vi "Engine In - Diesel - Sensors.vi"(0 "dt [sec]":sgl, 1 "ADCombo.Voltage [V]":sgl[](array[numeric]), 2 "ADCombo.Resistance [Ohm]":sgl[](array[numeric])) -> (8 "TDKBattV":sgl format="%0.2f", 9 "MAT [C]":sgl format="%0.2f", 10 "12VPulsBattV":sgl format="%0.2f", 11 "Oil Temp [C]":sgl, 12 "5VPulsBattV":sgl format="%0.2f", 13 "IAT [C]":sgl format="%0.2f", 14 "RailP [bar]":sgl format="%0.2f", 15 "ECT [C]":sgl format="%0.2f", 16 "Barometric Air Pressure [kPa]":sgl, 18 "Turbo Outlet Air Pressure [kPa]":sgl, 20 "MAP [kPa]":sgl format="%0.2f", 21 "Exhaust Manifold Pressure [kPa]":sgl, 22 "EGR DiffP [kPa]":sgl, 23 "Oil Pressure [kPa]":sgl, 24 "MAF [kg/hr]":sgl format="%0.2f", 25 "EGR Valve Position [%]":sgl, 26 "Pedal [%]":sgl format="%0.2f")   [LabVIEW 2015, in "ECS-RT.lvlib"]
uses:
  ECS-RT.lvlib
  <vilib>/ptbypt/NI_PtbyPt.lvlib
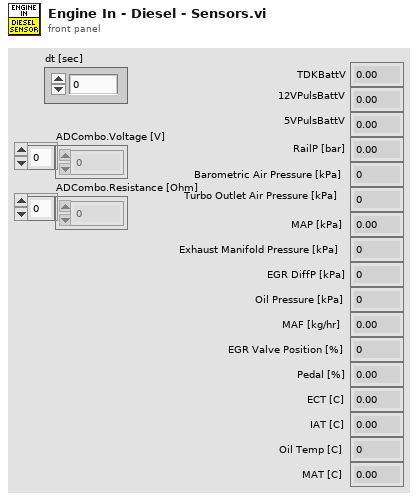
[diagram p1: front panel]
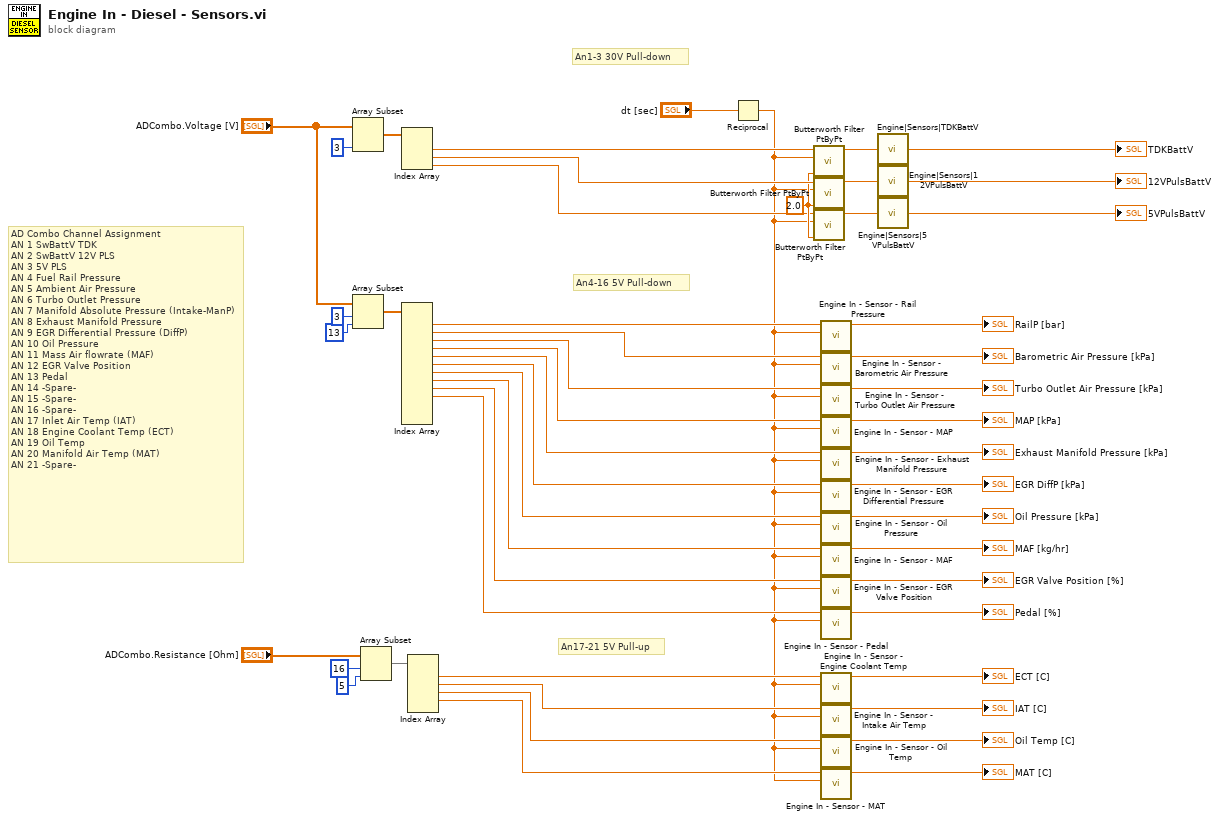
[diagram p0: block diagram]
diagram:
  w40 = 2.0 ("low cutoff freq: fl")
  # "An1-3 30V Pull-down"
  # "An17-21 5V Pull-up"
  # "An4-16 5V Pull-down"
  # "AD Combo Channel Assignment\nAN\t1\tSwBattV TDK\nAN\t2\tSwBattV 12V PLS\nAN\t3\t5V PLS\nAN\t4\tFuel Rail Pressure\nAN\t5\tAmbient Air Pressure\nAN\t6\tTurbo Outlet Pressure\nAN\t7\tManifold Absolute Pressure (Intake-ManP)\nAN\t8\tExhaust Manifold Pressure\nAN\t9\tEGR Differential Pressure (DiffP)\nAN\t10\tOil Pressure\nAN\t11\tMass Air flowrate (MAF)\nAN\t12\tEGR Valve Position\nAN\t13\tPedal\nAN\t14\t-Spare-\nAN\t15\t-Spare-\nAN\t16\t-Spare-\nAN\t17\tInlet Air Temp (IAT)\nAN\t18\tEngine Coolant Temp (ECT)\nAN\t19\tOil Temp\nAN\t20\tManifold Air Temp (MAT)\nAN\t21\t-Spare-"
  n1 = Array Subset(array="ADCombo.Voltage [V]", length=3) -> (w36:sgl[])  [unwired: 1 in]
  n2 = Array Subset(array="ADCombo.Voltage [V]", index=3, length=13) -> (w35:sgl[])
  n3 = Array Subset(array="ADCombo.Resistance [Ohm]", index=16, length=5) -> (w34:sgl[])
  n4 = Index Array(array=w36) -> (element #1=w43:sgl, element #2=w42:sgl, element #3=w14:sgl)  [unwired: 3 in]
  n5 = Index Array(array=w35) -> (element #1=w13:sgl, element #2=w12:sgl, element #3=w11:sgl, element #4=w10:sgl, element #5=w9:sgl, element #6=w8:sgl, element #7=w7:sgl, element #8=w6:sgl, element #9=w5:sgl, element #10=w4:sgl)  [unwired: 13 in, 3 out]
  n6 = Index Array(array=w34) -> (element #1=w3:sgl, element #2=w2:sgl, element #3=w29:sgl, element #4=w28:sgl)  [unwired: 5 in, 1 out]
  n7 = Reciprocal(x="dt [sec]") -> (1/x=w1:sgl)
  n8 = call <vilib>:"Butterworth Filter PtByPt.vi"("low cutoff freq: fl"=w40, "sampling freq: fs"=w1, "x"=w43) -> ("Filtered x"=w15:dbl)  [unwired: 4 in, 3 out]
  "TDKBattV" <- w15
  n9 = call <vilib>:"Butterworth Filter PtByPt.vi"("low cutoff freq: fl"=w40, "sampling freq: fs"=w1, "x"=w42) -> ("Filtered x"=w16:dbl)  [unwired: 4 in, 3 out]
  "12VPulsBattV" <- w16
  n10 = call <vilib>:"Butterworth Filter PtByPt.vi"("low cutoff freq: fl"=w40, "sampling freq: fs"=w1, "x"=w14) -> ("Filtered x"=w17:dbl)  [unwired: 4 in, 3 out]
  "5VPulsBattV" <- w17
  n11 = call "Engine In - Sensor - Rail Pressure.vi"("Loop Freq (Hz)"=w1, "Rail Pressure [V]"=w13) -> ("Rail Pressure [bar]"=→"RailP [bar]":sgl)  [unwired: 9 in]
  n12 = call "Engine In - Sensor - Barometric Air Pressure.vi"("Loop Freq (Hz)"=w1, "Barometric Air Pressure [V]"=w12) -> ("Barometric Air Pressure [kPa]"=→"Barometric Air Pressure [kPa]":sgl)  [unwired: 9 in]
  n13 = call "Engine In - Sensor - Turbo Outlet Air Pressure.vi"("Loop Freq (Hz)"=w1, "Turbo Outlet Air Pressure [V]"=w11) -> ("Turbo Outlet Air Pressure [kPa]"=→"Turbo Outlet Air Pressure [kPa]":sgl)  [unwired: 9 in]
  n14 = call "Engine In - Sensor - MAP.vi"("Loop Freq (Hz)"=w1, "Raw Intake Manifold Pressure [V]"=w10) -> ("Intake Manifold Pressure [kPa]"=→"MAP [kPa]":sgl)  [unwired: 9 in]
  n15 = call "Engine In - Sensor - Exhaust Manifold Pressure.vi"("Loop Freq (Hz)"=w1, "Exhaust Manifold Pressure [V]"=w9) -> ("Exhaust Manifold Pressure [kPa]"=→"Exhaust Manifold Pressure [kPa]":sgl)  [unwired: 9 in]
  n16 = call "Engine In - Sensor - EGR Differential Pressure.vi"("Loop Freq (Hz)"=w1, "EGR Differential Pressure [V]"=w8) -> ("EGR Differential Pressure [kPa]"=→"EGR DiffP [kPa]":sgl)  [unwired: 9 in]
  n17 = call "Engine In - Sensor - Oil Pressure.vi"("Loop Freq (Hz)"=w1, "Oil Pressure [V]"=w7) -> ("Oil Pressure [kPa]"=→"Oil Pressure [kPa]":sgl)  [unwired: 9 in]
  n18 = call "Engine In - Sensor - MAF.vi"("Loop Freq (Hz)"=w1, "MAF [V]"=w6) -> ("MAF [kg/hr]"=→"MAF [kg/hr]":sgl)  [unwired: 9 in]
  n19 = call "Engine In - Sensor - EGR Valve Position.vi"("Loop Freq (Hz)"=w1, "EGR Valve Position [V]"=w5) -> ("EGR Valve Position [%]"=→"EGR Valve Position [%]":sgl)  [unwired: 9 in]
  n20 = call "Engine In - Sensor - Pedal.vi"("Loop Freq (Hz)"=w1, "Pedal [V]"=w4) -> ("Pedal [%]"=→"Pedal [%]":sgl)  [unwired: 9 in]
  n21 = call "Engine In - Sensor - Engine Coolant Temp.vi"("Loop Freq [Hz]"=w1, "Engine Coolant Temp Raw [Ohm]"=w3) -> ("Engine Coolant Temp [C]"=→"ECT [C]":sgl)  [unwired: 9 in]
  n22 = call "Engine In - Sensor - Intake Air Temp.vi"("Loop Freq [Hz]"=w1, "Intake Air Temp Raw [Ohm]"=w2) -> ("Intake Air Temp [C]"=→"IAT [C]":sgl)  [unwired: 9 in]
  n23 = call "Engine In - Sensor - Oil Temp.vi"("Loop Freq [Hz]"=w1, "Oil Temp Raw [Ohm]"=w29) -> ("Oil Temp [C]"=→"Oil Temp [C]":sgl)  [unwired: 9 in]
  n24 = call "Engine In - Sensor - MAT.vi"("Loop Freq [Hz]"=w1, "Raw Intake Manifold Temp [Ohm]"=w28) -> ("Intake Manifold Temp [C]"=→"MAT [C]":sgl)  [unwired: 9 in]
  n25 = call "Engine|Sensors|TDKBattV"("Value"=w15) -> ()
  n26 = call "Engine|Sensors|12VPulsBattV"("Value"=w16) -> ()
  n27 = call "Engine|Sensors|5VPulsBattV"("Value"=w17) -> ()
